vi "Lin Verification Daten speichern.vi"(6 "Stufen Tabelle":T1, 9 "Lin Daten":T2 {"CalGas Eingang" items=["Cal Gas 1", "Cal Gas 2", "Cal Gas 3"]; "Max Fehler (Sollwert)" format="%#_5g"; "Zeitdauer Stufe" format="%#_5g"; "Anzahl Stufen" format="%#_5g"; "Verdünnungsgas" items=["N2", "O2"]}, 11 "Aktionen":T6) -> (0 "Stufen Tabellen":T1, 1 "Lin Daten Array":T2 {"CalGas Eingang" items=["Cal Gas 1", "Cal Gas 2", "Cal Gas 3"]; "Max Fehler (Sollwert)" format="%#_5g"; "Zeitdauer Stufe" format="%#_5g"; "Anzahl Stufen" format="%#_5g"; "Verdünnungsgas" items=["N2", "O2"]}, 3 "Gefunden?":bool)   [LabVIEW 2015, in "Linearisierung v2.lvlib" / "Linearity verification 1065-307.lvlib"]
uses:
  Linearity verification 1065-307.lvlib
  <vilib>/Utility/config.llb/NI_LVConfig.lvlib
  <vilib>/Utility/config.llb/Write Key (U32).vi
  <vilib>/Utility/config.llb/Write Key (String).vi
  Allgemein/allgemeine Sub-VIs.lvlib
  <vilib>/Utility/config.llb/Read Key (U32).vi
  <vilib>/Utility/config.llb/Write Key (Double).vi
  <vilib>/Utility/config.llb/Read Key (String).vi
  <vilib>/Utility/config.llb/Read Key (Double).vi
  Visualisierungs Elemente/String - Eingabefeld.ctl
  Visualisierungs Elemente/Zahlen-Eingabefeld.ctl
  Gasteiler/Lin Daten.ctl
  Gasteiler/Gasteiler.lvlib
  Gasteiler/Stufen Tabelle.ctl
  Seiten/FT-IR/FT-IR.lvlib
  Seiten/FT-IR/FGV FT-IR Gasliste Aktionen.ctl
  Messdaten/Messdaten.lvlib
  Messdaten/Aktionen FGV Messdaten.ctl
  LinVer Daten verwalten Aktionen.ctl
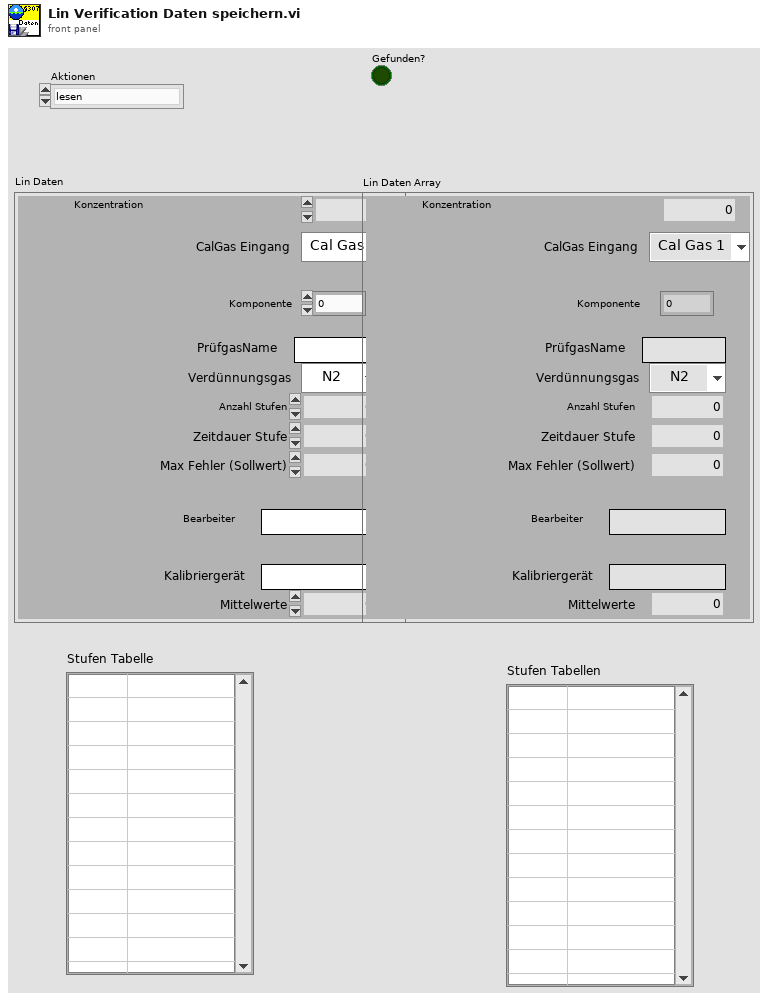
[diagram p1: front panel]
types:
  T1 = typedef "Linearisierung v2.lvlib/Gasteiler.lvlib/Stufen Tabelle.ctl" = string[][]
  T2 = typedef "Linearisierung v2.lvlib/Gasteiler.lvlib/Lin Daten.ctl" = cluster{"PrüfgasName":T3, "Verdünnungsgas":T4, "Anzahl Stufen":T5, "Zeitdauer Stufe":T5, "Max Fehler (Sollwert)":T5, "Bearbeiter":T3, "Kalibriergerät":T3, "Mittelwerte":i32, "Komponente":u16, "CalGas Eingang":u16, "Konzentration":sgl}
  T3 = typedef "String - Eingabefeld.ctl" = string
  T4 = typedef "Linearisierung v2.lvlib/Gasteiler.lvlib/Prüfgas in.ctl" = u16
  T5 = typedef "Zahlen-Eingabefeld.ctl" = sgl
  T6 = typedef "Linearisierung v2.lvlib/Linearity verification 1065-307.lvlib/LinVer Daten verwalten Aktionen.ctl" = enum16{"lesen", "speichern", "laden", "Lin Daten schr.", "Stufen Tabelle", "Lin Name AK", "Lin Pfad AK"}
  T7 = typedef "Messdaten.lvlib/Aktionen FGV Messdaten.ctl" = enum16{"lesen", "schreiben", "löschen", "Mittelwerte", "Komponente"}
  T8 = typedef "FT-IR.lvlib/FGV FT-IR Gasliste Aktionen.ctl" = enum16{"lesen", "Gasliste FT-IR", "Gasliste ausgelesen", "laden", "speichern", "löschen"}
  T9 = typedef "String - Ausgabefeld.ctl" = string
  T10 = typedef "NI_LVConfig.lvlib/Config Data RefNum.ctl" = refnum<k1>
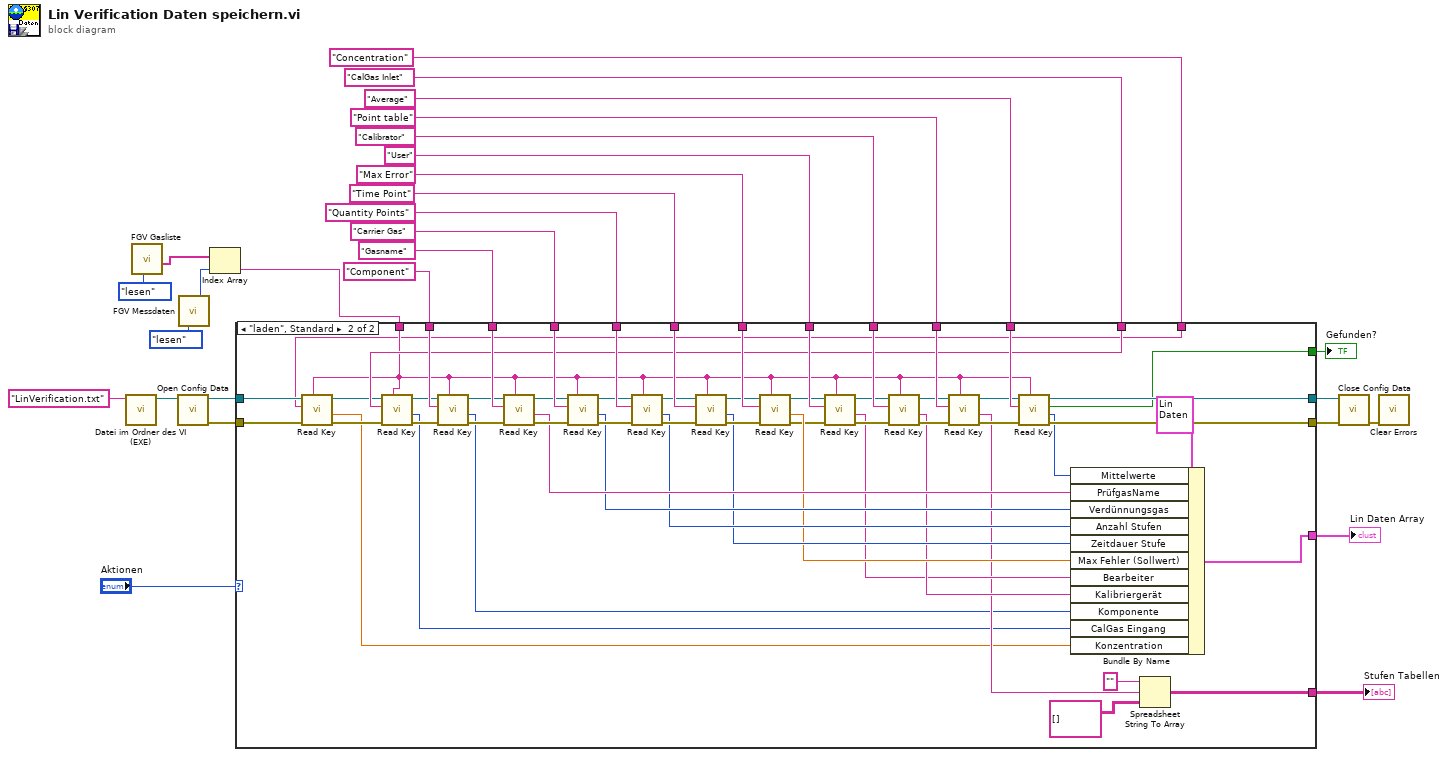
[diagram p0: block diagram]
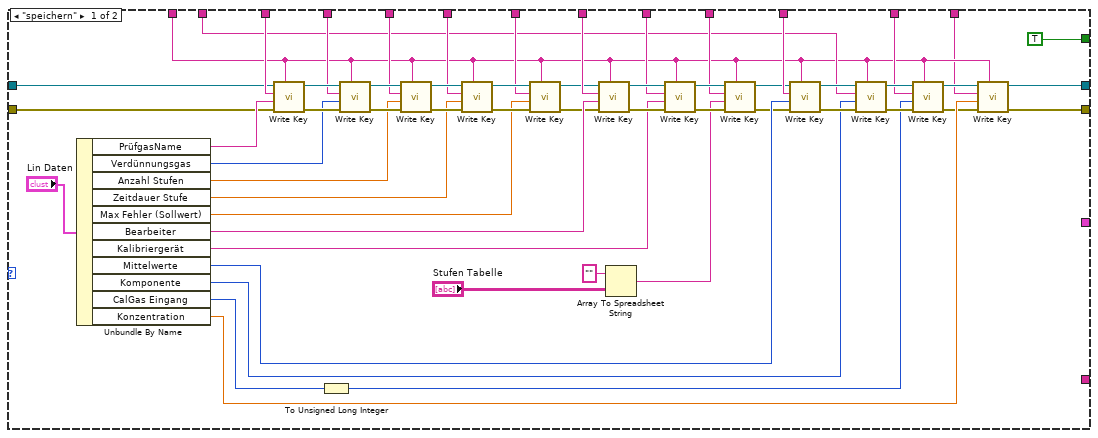
[diagram p2: hidden frame]
diagram:
  n1 = call "Datei im Ordner des VI (EXE).vi"("Dateiname"="LinVerification.txt") -> ("Dateipfad im Ordner des Haupt-VIs"=w28:path)  [unwired: 8 in, 2 out]
  n2 = call "FGV Gasliste.vi"("Aktionen"=FGV_FT-IR_Gasliste_Aktionen."lesen") -> ("Aktuelle Gasliste gesamt"=w5:T9[])  [unwired: 8 in, 2 out]
  n3 = call <vilib>:"Open Config Data.vi"("configuration file path"=w28) -> ("error out"=w25:errorcluster, "refnum"=w26:T10)  [unwired: 8 in, 1 out]
  n4 = call "FGV Messdaten.vi"("Aktionen"=Aktionen_FGV_Messdaten."lesen") -> ("Komponente"=w3:u16)  [unwired: 6 in, 8 out]
  n5 = Index Array(array=w5, index=w3) -> (element=w2:T9)
  n6 = case shown="\"laden\", Standard" "Aktionen" {
    tunnel: w26 -> [w51 w92]
    tunnel: w25 -> [w50 w91]
    tunnel: [w33 w141] -> w24
    tunnel: [w32 w140] -> w23
    tunnel: "Gasname" ("key") -> [w68 w139]
    tunnel: "Carrier Gas" ("key") -> [w67 w138]
    tunnel: "Quantity Points" ("key") -> [w66 w137]
    tunnel: "Time Point" ("key") -> [w65 w136]
    tunnel: "Max Error" ("key") -> [w64 w135]
    tunnel: "User" ("key") -> [w63 w134]
    tunnel: "Calibrator" ("key") -> [w62 w133]
    tunnel: w2 -> [w31 w88]
    tunnel: "Point table" ("key") -> [w58 w132]
    tunnel: "Average" ("key") -> [w53 w130]
    tunnel: [_ w131] -> w11
    tunnel: [_ w102] -> w10
    tunnel: "Component" ("key") -> [w43 w98]
    tunnel: "CalGas Inlet" ("key") -> [w38 w94]
    tunnel: "Concentration" ("key") -> [w30 w87]
    tunnel: [TRUE w85] -> w1
    frame "speichern" {
      n7 = Unbundle By Name("Lin Daten") -> ("PrüfgasName"=w73:T3, "Verdünnungsgas"=w72:T4, "Anzahl Stufen"=w71:T5, "Zeitdauer Stufe"=w70:T5, "Max Fehler (Sollwert)"=w69:T5, "Bearbeiter"=w55:T3, "Kalibriergerät"=w54:T3, "Mittelwerte"=w52:i32, "Komponente"=w42:u16, "CalGas Eingang"=w39:u16, "Konzentration"=w36:sgl)
      n8 = call-poly <vilib>:"Write Key.vi"("section"=w31, "error in (no error)"=w50, "value"=w73, "key"=w68, "refnum"=w51) -> ("error out"=w84:errorcluster, "refnum out"=w83:T10)  [unwired: 4 in, 1 out]
      n9 = To Unsigned Long Integer(number=w39) -> (unsigned 32bit integer=w37:u32)
      n10 = call-poly <vilib>:"Write Key.vi"("section"=w31, "error in (no error)"=w84, "value"=w72, "key"=w67, "refnum"=w83) -> ("error out"=w82:errorcluster, "refnum out"=w81:T10)  [unwired: 4 in, 1 out]
      n11 = call-poly <vilib>:"Write Key.vi"("section"=w31, "error in (no error)"=w82, "value"=w71, "key"=w66, "refnum"=w81) -> ("error out"=w76:errorcluster, "refnum out"=w79:T10)  [unwired: 4 in, 1 out]
      n12 = call-poly <vilib>:"Write Key.vi"("section"=w31, "error in (no error)"=w76, "value"=w70, "key"=w65, "refnum"=w79) -> ("error out"=w75:errorcluster, "refnum out"=w78:T10)  [unwired: 4 in, 1 out]
      n13 = call-poly <vilib>:"Write Key.vi"("section"=w31, "error in (no error)"=w75, "value"=w69, "key"=w64, "refnum"=w78) -> ("error out"=w48:errorcluster, "refnum out"=w49:T10)  [unwired: 4 in, 1 out]
      n14 = call-poly <vilib>:"Write Key.vi"("section"=w31, "error in (no error)"=w48, "value"=w55, "key"=w63, "refnum"=w49) -> ("error out"=w74:errorcluster, "refnum out"=w77:T10)  [unwired: 4 in, 1 out]
      n15 = Array To Spreadsheet String(array="Stufen Tabelle", 3:"" ("Format-String")) -> (spreadsheet string=w57:string)  [unwired: 1 in]
      n16 = call-poly <vilib>:"Write Key.vi"("section"=w31, "error in (no error)"=w74, "value"=w54, "key"=w62, "refnum"=w77) -> ("error out"=w59:errorcluster, "refnum out"=w60:T10)  [unwired: 4 in, 1 out]
      n17 = call-poly <vilib>:"Write Key.vi"("section"=w31, "error in (no error)"=w59, "value"=w57, "key"=w58, "refnum"=w60) -> ("error out"=w46:errorcluster, "refnum out"=w47:T10)  [unwired: 4 in, 1 out]
      n18 = call-poly <vilib>:"Write Key.vi"("section"=w31, "error in (no error)"=w46, "value"=w52, "key"=w53, "refnum"=w47) -> ("error out"=w44:errorcluster, "refnum out"=w45:T10)  [unwired: 4 in, 1 out]
      n19 = call-poly <vilib>:"Write Key.vi"("section"=w31, "error in (no error)"=w44, "value"=w42, "key"=w43, "refnum"=w45) -> ("error out"=w41:errorcluster, "refnum out"=w40:T10)  [unwired: 4 in, 1 out]
      n20 = call-poly <vilib>:"Write Key.vi"("section"=w31, "error in (no error)"=w41, "value"=w37, "key"=w38, "refnum"=w40) -> ("error out"=w35:errorcluster, "refnum out"=w34:T10)  [unwired: 4 in, 1 out]
      n21 = call-poly <vilib>:"Write Key.vi"("section"=w31, "error in (no error)"=w35, "value"=w36, "key"=w30, "refnum"=w34) -> ("error out"=w32:errorcluster, "refnum out"=w33:T10)  [unwired: 4 in, 1 out]
    }
    frame "laden", Default {
      n22 = call-poly <vilib>:"Read Key.vi"("section"=w88, "error in (no error)"=w91, "key"=w87, "refnum"=w92) -> ("error out"=w90:errorcluster, "value"=w86:dbl, "refnum out"=w89:T10)  [unwired: 4 in, 1 out]
      n23 = call-poly <vilib>:"Read Key.vi"("section"=w88, "error in (no error)"=w90, "key"=w94, "refnum"=w89) -> ("error out"=w95:errorcluster, "value"=w93:u32, "refnum out"=w96:T10)  [unwired: 4 in, 1 out]
      n24 = call-poly <vilib>:"Read Key.vi"("section"=w88, "error in (no error)"=w95, "key"=w98, "refnum"=w96) -> ("error out"=w99:errorcluster, "value"=w97:u32, "refnum out"=w100:T10)  [unwired: 4 in, 1 out]
      n25 = call-poly <vilib>:"Read Key.vi"("section"=w88, "error in (no error)"=w99, "key"=w139, "refnum"=w100) -> ("error out"=w128:errorcluster, "value"=w118:string, "refnum out"=w129:T10)  [unwired: 4 in, 1 out]
      n26 = call-poly <vilib>:"Read Key.vi"("section"=w88, "error in (no error)"=w128, "key"=w138, "refnum"=w129) -> ("error out"=w126:errorcluster, "value"=w117:u32, "refnum out"=w127:T10)  [unwired: 4 in, 1 out]
      n27 = call-poly <vilib>:"Read Key.vi"("section"=w88, "error in (no error)"=w126, "key"=w137, "refnum"=w127) -> ("error out"=w124:errorcluster, "value"=w116:u32, "refnum out"=w125:T10)  [unwired: 4 in, 1 out]
      n28 = call-poly <vilib>:"Read Key.vi"("section"=w88, "error in (no error)"=w124, "key"=w136, "refnum"=w125) -> ("error out"=w122:errorcluster, "value"=w115:u32, "refnum out"=w123:T10)  [unwired: 4 in, 1 out]
      n29 = call-poly <vilib>:"Read Key.vi"("section"=w88, "error in (no error)"=w122, "key"=w135, "refnum"=w123) -> ("error out"=w107:errorcluster, "value"=w114:dbl, "refnum out"=w108:T10)  [unwired: 4 in, 1 out]
      n30 = call-poly <vilib>:"Read Key.vi"("section"=w88, "error in (no error)"=w107, "key"=w134, "refnum"=w108) -> ("error out"=w120:errorcluster, "value"=w110:string, "refnum out"=w121:T10)  [unwired: 4 in, 1 out]
      n31 = call-poly <vilib>:"Read Key.vi"("section"=w88, "error in (no error)"=w120, "key"=w133, "refnum"=w121) -> ("error out"=w113:errorcluster, "value"=w111:string, "refnum out"=w112:T10)  [unwired: 4 in, 1 out]
      n32 = call-poly <vilib>:"Read Key.vi"("section"=w88, "error in (no error)"=w113, "key"=w132, "refnum"=w112) -> ("error out"=w105:errorcluster, "value"=w104:string, "refnum out"=w106:T10)  [unwired: 4 in, 1 out]
      n33 = call-poly <vilib>:"Read Key.vi"("section"=w88, "error in (no error)"=w105, "key"=w130, "refnum"=w106) -> ("error out"=w140:errorcluster, "value"=w109:u32, "found?"=w85:bool, "refnum out"=w141:T10)  [unwired: 4 in]
      n34 = Bundle By Name(cluster=T2 {"PrüfgasName"="", "Verdünnungsgas"=0, "Anzahl Stufen"=0.0, "Zeitdauer Stufe"=0.0, "Max Fehler (Sollwert)"=0.0, "Bearbeiter"="", "Kalibriergerät"="", "Mittelwerte"=0, "Komponente"=0, "CalGas Eingang"=0, "Konzentration"=0.0} ("Lin Daten"), "Mittelwerte"=w109, "PrüfgasName"=w118, "Verdünnungsgas"=w117, "Anzahl Stufen"=w116, "Zeitdauer Stufe"=w115, "Max Fehler (Sollwert)"=w114, "Bearbeiter"=w110, "Kalibriergerät"=w111, "Komponente"=w97, "CalGas Eingang"=w93, "Konzentration"=w86) -> (w131:T2)
      n35 = Spreadsheet String To Array(format string="" ("Format-String"), spreadsheet string=w104, array type (2D Dbl)=T1 [] ("Stufen Tabelle")) -> (array=w102:string[][])  [unwired: 1 in]
    }
  }
  "Lin Daten Array" <- w11
  "Stufen Tabellen" <- w10
  "Gefunden?" <- w1
  n36 = call <vilib>:"Close Config Data.vi"("error in (no error)"=w23, "refnum"=w24) -> ("error out"=w14:errorcluster)  [unwired: 8 in, 1 out]
  n37 = call <vilib>:"Clear Errors.vi"("error in (no error)"=w14) -> ()  [unwired: 5 in, 2 out]
